vi "DRC Write Set Point.vi"(0 "Set Point":dbl=0.1 format="%.2f", 1 "VISA session":refnum<visa-resource-name>) -> ()   [LabVIEW 2021]
doc: "This VI reads the setpoint from a Lakeshore DRC 93C or 82C temperature controller, increments it by the specified amount and sends it back.\nScott Hannahs, FBNML May 1991"
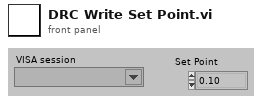
[diagram p1: front panel]
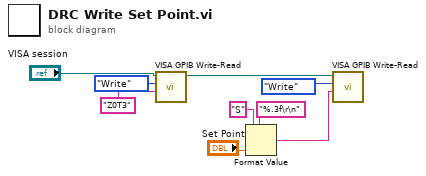
[diagram p0: block diagram]
diagram:
  n1 = call "VISA GPIB Write-Read.vi"("Command"="Z0T3", "Action"=enum16{"Write", "Read", "Write & Read"}."Write", "VISA resource name"="VISA session") -> ("dup VISA Session"=w5:refnum<visa-resource-name>)  [unwired: 5 in, 3 out]
  n2 = Format Value(string ("")="S", format string="%.3f\r\n", value (0)="Set Point") -> (output string=w6:string)
  n3 = call "VISA GPIB Write-Read.vi"("Command"=w6, "Action"=enum16{"Write", "Read", "Write & Read"}."Write", "VISA resource name"=w5) -> ()  [unwired: 5 in, 4 out]
